vi "Read URL.vi"(8 "error in (no error)":errorcluster, 11 "SQS in":refnum<class "Queue.lvclass">) -> (0 "error out":errorcluster, 2 "URL":string, 3 "SQS out":refnum<class "Queue.lvclass">)   [LabVIEW 2015, in "NI_AWS_SQS.lvlib" / "Queue.lvclass"]
uses:
  Queue.lvclass
  Queue.lvclass/Queue.ctl
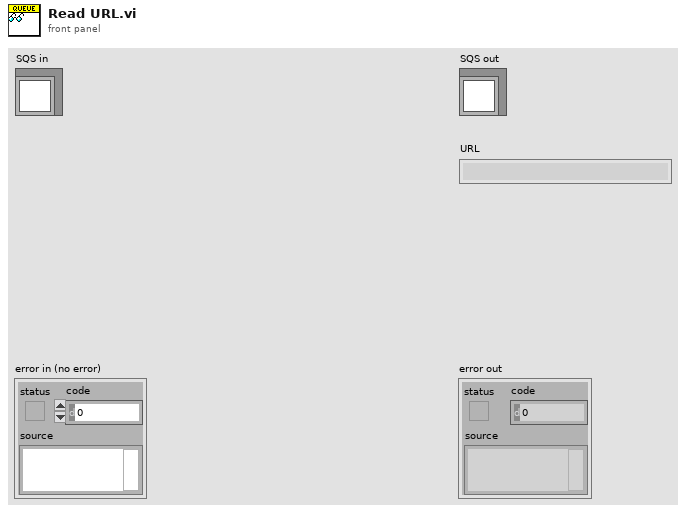
[diagram p1: front panel]
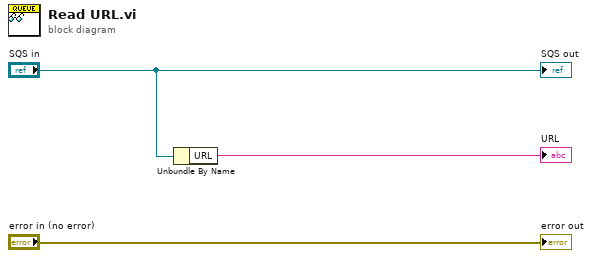
[diagram p0: block diagram]
diagram:
  n1 = Unbundle By Name("SQS in") -> ("URL"=→"URL":string)
  "error out" <- "error in (no error)"
  "SQS out" <- "SQS in"
